vi "rszvl_core_global.vi"() -> ()   [LabVIEW 2014] (continued)
 Callback"="", "Supported Models"="", "Instrument Options"="", "Repeated Capabilities"="", "Restricted Repeated Capabilities"="", "Help"="This attribute switches measurements with a power sensor on or off.\n\nAvailable Repeated Capabilities:\nNone\n\nRemote-control command(s):\n[SENSe<1|2>:]PMETer[:STATe] ON | OFF", "Flags"={"OPC Wait"=FALSE, "Dont check status"=FALSE, "*WAI"=FALSE}, "Check Status Callback"=""}, {"Level"=3, "Descriptive Name"="PWM Averaging State", "Class Only"=FALSE, "Data Type"=3, "Access"=2, "Identifier"="RSZVL_ATTR_PMET_AVERAGE_AUTO", "Range Table"="", "Command"="SENS:PMET:MTIM:AVER:STAT", "Read Callback"="", "Write Callback"="", "Range Callback"="", "Check Callback"="", "Rngtable Callback"="", "Coerce Callback"="", "User Callback"="", "Supported Models"="", "Instrument Options"="", "Repeated Capabilities"="", "Restricted Repeated Capabilities"="", "Help"="This attribute activates or deactivates manual averaging. The average count is set with the [SENSe<1|2>:]PMETer:MTIMe:AVERage:COUNt command (RSZVL_ATTR_PMET_AVERAGE_COUNT attribute).\n\nAvailable Repeated Capabilities:\nNone\n\nRemote-control command(s):\n[SENSe<1|2>:]PMETer:MTIMe:AVERage[:STATe] ON | OFF", "Flags"={"OPC Wait"=FALSE, "Dont check status"=FALSE, "*WAI"=FALSE}, "Check Status Callback"=""}, {"Level"=3, "Descriptive Name"="PWM Averaging Count", "Class Only"=FALSE, "Data Type"=0, "Access"=2, "Identifier"="RSZVL_ATTR_PMET_AVERAGE_COUNT", "Range Table"="rszvl_rngPmetAverCount", "Command"="SENS:PMET:MTIM:AVER:COUN", "Read Callback"="", "Write Callback"="", "Range Callback"="", "Check Callback"="", "Rngtable Callback"="", "Coerce Callback"="", "User Callback"="", "Supported Models"="", "Instrument Options"="", "Repeated Capabilities"="", "Restricted Repeated Capabilities"="", "Help"="This attribute defines the number of readings (averagings) to be performed after a single sweep has been started. This attribute is only available if the [SENSe<1|2>:]PMETer:MTIMe:AVERage[:STATe] command (RSZVL_ATTR_PMET_AVERAGE_AUTO attribute) is set to ON. Results become more stable with extended average, particularly if signals with low power are measured. This setting can be used to minimize the influence of noise in the power meter measurement.\n\nAvailable Repeated Capabilities:\nNone\n\nRemote-control command(s):\n[SENSe<1|2>:]PMETer:MTIMe:AVERage:COUNt", "Flags"={"OPC Wait"=FALSE, "Dont check status"=FALSE, "*WAI"=FALSE}, "Check Status Callback"=""}, {"Level"=3, "Descriptive Name"="PWM Reference Level Offset State", "Class Only"=FALSE, "Data Type"=3, "Access"=2, "Identifier"="RSZVL_ATTR_PMET_REF_LEVEL_OFFSET_STATE", "Range Table"="", "Command"="SENS:PMET:ROFF:STAT", "Read Callback"="", "Write Callback"="", "Range Callback"="", "Check Callback"="", "Rngtable Callback"="", "Coerce Callback"="", "User Callback"="", "Supported Models"="", "Instrument Options"="", "Repeated Capabilities"="", "Restricted Repeated Capabilities"="", "Help"="This attribute defines whether the reference level offset set for the analyzer is taken into account for the measured power or not.\n\nAvailable Repeated Capabilities:\nNone\n\nRemote-control command(s):\n[SENSe<1|2>:]PMETer:ROFFset[:STATe] ON | OFF", "Flags"={"OPC Wait"=FALSE, "Dont check status"=FALSE, "*WAI"=FALSE}, "Check Status Callback"=""}, {"Level"=2, "Descriptive Name"="Display", "Class Only"=TRUE, "Data Type"=0, "Access"=0, "Identifier"="", "Range Table"="", "Command"="", "Read Callback"="", "Write Callback"="", "Range Callback"="", "Check Callback"="", "Rngtable Callback"="", "Coerce Callback"="", "User Callback"="", "Supported Models"="", "Instrument Options"="", "Repeated Capabilities"="", "Restricted Repeated Capabilities"="", "Help"="(1) PWM Result Display:\nThis attribute switches bargraph display on or off for measurements with a power sensor. If bargraph display is switched off, the measurement value appears in the Marker Info field.\n\n(2) PWM Rel/Abs Display:\nThis attribute switches between relative and absolute display of the result.", "Flags"={"OPC Wait"=FALSE, "Dont check status"=FALSE, "*WAI"=FALSE}, "Check Status Callback"=""}, {"Level"=3, "Descriptive Name"="PWM Rel/Abs Display", "Class Only"=FALSE, "Data Type"=3, "Access"=2, "Identifier"="RSZVL_ATTR_PMET_RELATIVE", "Range Table"="", "Command"="CALC:PMET:REL:STAT", "Read Callback"="", "Write Callback"="", "Range Callback"="", "Check Callback"="", "Rngtable Callback"="", "Coerce Callback"="", "User Callback"="", "Supported Models"="", "Instrument Options"="", "Repeated Capabilities"="", "Restricted Repeated Capabilities"="", "Help"="This attribute switches between relative and absolute display of the result.\n\nAvailable Repeated Capabilities:\nNone\n\nRemote-control command(s):\nCALCulate<1|2>:PMETer:RELative:STATe ON | OFF", "Flags"={"OPC Wait"=FALSE, "Dont check status"=FALSE, "*WAI"=FALSE}, "Check Status Callback"=""}, {"Level"=2, "Descriptive Name"="Results", "Class Only"=TRUE, "Data Type"=0, "Access"=0, "Identifier"="", "Range Table"="", "Command"="", "Read Callback"="", "Write Callback"="", "Range Callback"="", "Check Callback"="", "Rngtable Callback"="", "Coerce Callback"="", "User Callback"="", "Supported Models"="", "Instrument Options"="", "Repeated Capabilities"="", "Restricted Repeated Capabilities"="", "Help"="(1) PWM Read Result:\nThis attribute triggers a measurement with the power sensor and then outputs the result.\n\n(2) PWM Fetch Result:\nThis attribute outputs the result of the power sensor.", "Flags"={"OPC Wait"=FALSE, "Dont check status"=FALSE, "*WAI"=FALSE}, "Check Status Callback"=""}, {"Level"=3, "Descriptive Name"="PWM Read Result", "Class Only"=FALSE, "Data Type"=1, "Access"=0, "Identifier"="RSZVL_ATTR_PMET_READ", "Range Table"="", "Command"="READ:PMET?", "Read Callback"="", "Write Callback"="", "Range Callback"="", "Check Callback"="", "Rngtable Callback"="", "Coerce Callback"="", "User Callback"="", "Supported Models"="", "Instrument Options"="", "Repeated Capabilities"="", "Restricted Repeated Capabilities"="", "Help"="This attribute triggers a measurement with the power sensor and then outputs the result.\n\nAvailable Repeated Capabilities:\nNone\n\nRemote-control command(s):\nREAD<1|2>:PMETer?", "Flags"={"OPC Wait"=TRUE, "Dont check status"=FALSE, "*WAI"=FALSE}, "Check Status Callback"=""}, {"Level"=3, "Descriptive Name"="PWM Fetch Result", "Class Only"=FALSE, "Data Type"=1, "Access"=0, "Identifier"="RSZVL_ATTR_PMET_FETCH", "Range Table"="", "Command"="FETC:PMET?", "Read Callback"="", "Write Callback"="", "Range Callback"="", "Check Callback"="", "Rngtable Callback"="", "Coerce Callback"="", "User Callback"="", "Supported Models"="", "Instrument Options"="", "Repeated Capabilities"="", "Restricted Repeated Capabilities"="", "Help"="This attribute outputs the result of the power sensor.\n\nAvailable Repeated Capabilities:\nNone\n\nRemote-control command(s):\nFETCh<1|2>:PMETer?", "Flags"={"OPC Wait"=FALSE, "Dont check status"=FALSE, "*WAI"=FALSE}, "Check Status Callback"=""}, {"Level"=1, "Descriptive Name"="K14 - Spectrogram Measurement", "Class Only"=TRUE, "Data Type"=0, "Access"=0, "Identifier"="", "Range Table"="", "Command"="", "Read Callback"="", "Write Callback"="", "Range Callback"="", "Check Callback"="", "Rngtable Callback"="", "Coerce Callback"="", "User Callback"="", "Supported Models"="", "Instrument Options"="", "Repeated Capabilities"="", "Restricted Repeated Capabilities"="", "Help"="This class contains attributes for the Spectrogram Measurement option (K14).\n\n(1) Settings (Class):\nAttributes that configure Spectrogram.\n\n(2) Marker Settings (Class):\nAttributes that configure markers for Spectrogram.", "Flags"={"OPC Wait"=FALSE, "Dont check status"=FALSE, "*WAI"=FALSE}, "Check Status Callback"=""}, {"Level"=2, "Descriptive Name"="Settings", "Class Only"=TRUE, "Data Type"=0, "Access"=0, "Identifier"="", "Range Table"="", "Command"="", "Read Callback"="", "Write Callback"="", "Range Callback"="", "Check Callback"="", "Rngtable Callback"="", "Coerce Callback"="", "User Callback"="", "Supported Models"="", "Instrument Options"="", "Repeated Capabilities"="", "Restricted Repeated Capabilities"="", "Help"="Attributes that configure Spectrogram.\n\n(1) Spectrogram State:\nThis attribute activates or deactivates the Spectrogram Measurement option.\n\n(2) Spectrogram Color:\nThis attribute defines the frame color setting.\n\n(3) Spectrogram Display Size:\nThis attribute changes the screen layout.\n\n(4) Spectrogram History Buffer:\nThis attribute sets the number of frames to be stored in the history buffer.\n\n(5) Spectrogram Time Stamp:\nThis attribute activates or deactivates the time stamp.\n\n(6) Spectrogram Frame Count:\nThis attribute sets the number of frames recorded in a single sweep measurement.\n\n(7) Spectrogram Frame Select:\nThis attribute selects the frame if no measurement is running. During a measurement, the value is fixed to 0 and this command is not available.\n\n(8) Spectrogram Continue Frame:\nThis attribute determines whether the results of the last measurement are deleted before starting a new measurement in single sweep mode.\n\n(9) Spectrogram Clear:\nThis attribute deletes the spectrogram result display and the history buffer.\n\n(10) Spectrogram File Items to Save Recall Spectrogram:\nThis attribute adds the spectrogram data to the list of data subsets of a save/recall device setting.", "Flags"={"OPC Wait"=FALSE, "Dont check status"=FALSE, "*WAI"=FALSE}, "Check Status Callback"=""}, {"Level"=3, "Descriptive Name"="Spectrogram State", "Class Only"=FALSE, "Data Type"=3, "Access"=2, "Identifier"="RSZVL_ATTR_SPEM_STATE", "Range Table"="", "Command"="CALC:SPEC", "Read Callback"="", "Write Callback"="", "Range Callback"="", "Check Callback"="", "Rngtable Callback"="", "Coerce Callback"="", "User Callback"="", "Supported Models"="", "Instrument Options"="", "Repeated Capabilities"="", "Restricted Repeated Capabilities"="", "Help"="This attribute activates or deactivates the Spectrogram Measurement option.\n\nAvailable Repeated Capabilities:\nNone\n\nRemote-control command(s):\nCALCulate<1|2>:SPECtrogram[:STATe] OFF | ON", "Flags"={"OPC Wait"=FALSE, "Dont check status"=FALSE, "*WAI"=FALSE}, "Check Status Callback"=""}, {"Level"=3, "Descriptive Name"="Spectrogram Color", "Class Only"=FALSE, "Data Type"=0, "Access"=2, "Identifier"="RSZVL_ATTR_SPEM_COLOR", "Range Table"="rszvl_rngSpemColor", "Command"="CALC:SPEC:COL", "Read Callback"="", "Write Callback"="", "Range Callback"="", "Check Callback"="", "Rngtable Callback"="", "Coerce Callback"="", "User Callback"="", "Supported Models"="", "Instrument Options"="", "Repeated Capabilities"="", "Restricted Repeated Capabilities"="", "Help"="This attribute defines the frame color setting.\n\nAvailable Repeated Capabilities:\nNone\n\nRemote-control command(s):\nCALCulate<1|2>:SPECtrogram:COLor", "Flags"={"OPC Wait"=FALSE, "Dont check status"=FALSE, "*WAI"=FALSE}, "Check Status Callback"=""}, {"Level"=3, "Descriptive Name"="Spectrogram Display Size", "Class Only"=FALSE, "Data Type"=0, "Access"=2, "Identifier"="RSZVL_ATTR_SPEM_SIZE", "Range Table"="rszvl_rngDISPSizeWindow", "Command"="CALC:SPEC:SIZE", "Read Callback"="", "Write Callback"="", "Range Callback"="", "Check Callback"="", "Rngtable Callback"="", "Coerce Callback"="", "User Callback"="", "Supported Models"="", "Instrument Options"="", "Repeated Capabilities"="", "Restricted Repeated Capabilities"="", "Help"="This attribute changes the screen layout.\n\nAvailable Repeated Capabilities:\nNone\n\nRemote-control command(s):\nCALCulate<1|2>:SPECtrogram:SIZE", "Flags"={"OPC Wait"=FALSE, "Dont check status"=FALSE, "*WAI"=FALSE}, "Check Status Callback"=""}, {"Level"=3, "Descriptive Name"="Spectrogram History Buffer", "Class Only"=FALSE, "Data Type"=0, "Access"=2, "Identifier"="RSZVL_ATTR_SPEM_HDEP", "Range Table"="rszvl_rngSpemHistoryBuffDepth", "Command"="CALC:SPEC:HDEP", "Read Callback"="", "Write Callback"="", "Range Callback"="", "Check Callback"="", "Rngtable Callback"="", "Coerce Callback"="", "User Callback"="", "Supported Models"="", "Instrument Options"="", "Repeated Capabilities"="", "Restricted Repeated Capabilities"="", "Help"="This attribute sets the number of frames to be stored in the history buffer.\n\nAvailable Repeated Capabilities:\nNone\n\nRemote-control command(s):\nCALCulate<1|2>:SPECtrogram:HDEPth", "Flags"={"OPC Wait"=FALSE, "Dont check status"=FALSE, "*WAI"=FALSE}, "Check Status Callback"=""}, {"Level"=3, "Descriptive Name"="Spectrogram Time Stamp", "Class Only"=FALSE, "Data Type"=3, "Access"=2, "Identifier"="RSZVL_ATTR_SPEM_TIME_STAMP_STATE", "Range Table"="", "Command"="CALC:SPEC:TST", "Read Callback"="", "Write Callback"="", "Range Callback"="", "Check Callback"="", "Rngtable Callback"="", "Coerce Callback"="", "User Callback"="", "Supported Models"="", "Instrument Options"="", "Repeated Capabilities"="", "Restricted Repeated Capabilities"="", "Help"="This attribute activates or deactivates the time stamp.\n\nAvailable Repeated Capabilities:\nNone\n\nRemote-control command(s):\nCALCulate<1|2>:SPECtrogram:TSTamp[:STATe]", "Flags"={"OPC Wait"=FALSE, "Dont check status"=FALSE, "*WAI"=FALSE}, "Check Status Callback"=""}, {"Level"=3, "Descriptive Name"="Spectrogram Frame Count", "Class Only"=FALSE, "Data Type"=0, "Access"=2, "Identifier"="RSZVL_ATTR_SPEM_FRAME_COUNT", "Range Table"="", "Command"="CALC:SPEC:FRAM:COUN", "Read Callback"="", "Write Callback"="", "Range Callback"="", "Check Callback"="", "Rngtable Callback"="", "Coerce Callback"="", "User Callback"="", "Supported Models"="", "Instrument Options"="", "Repeated Capabilities"="", "Restricted Repeated Capabilities"="", "Help"="This attribute sets the number of frames recorded in a single sweep measurement.\n\nAvailable Repeated Capabilities:\nNone\n\nRemote-control command(s):\nCALCulate<1|2>:SPECtrogram:FRAMe:COUNt", "Flags"={"OPC Wait"=FALSE, "Dont check status"=FALSE, "*WAI"=FALSE}, "Check Status Callback"=""}, {"Level"=3, "Descriptive Name"="Spectrogram Frame Select", "Class Only"=FALSE, "Data Type"=0, "Access"=2, "Identifier"="RSZVL_ATTR_SPEM_FRAME_SELECT", "Range Table"="", "Command"="CALC:SPEC:FRAM:SEL", "Read Callback"="", "Write Callback"="", "Range Callback"="", "Check Callback"="", "Rngtable Callback"="", "Coerce Callback"="", "User Callback"="", "Supported Models"="", "Instrument Options"="", "Repeated Capabilities"="", "Restricted Repeated Capabilities"="", "Help"="This attribute selects the frame if no measurement is running. During a measurement, the value is fixed to 0 and this command is not available.\n\nAvailable Repeated Capabilities:\nNone\n\nRemote-control command(s):\nCALCulate<1|2>:SPECtrogram:FRAMe:SELect", "Flags"={"OPC Wait"=FALSE, "Dont check status"=FALSE, "*WAI"=FALSE}, "Check Status Callback"=""}, {"Level"=3, "Descriptive Name"="Spectrogram Continue Frame", "Class Only"=FALSE, "Data Type"=3, "Access"=2, "Identifier"="RSZVL_ATTR_SPEM_CONTINUOUS", "Range Table"="", "Command"="CALC:SPEC:CONT", "Read Callback"="", "Write Callback"="", "Range Callback"="", "Check Callback"="", "Rngtable Callback"="", "Coerce Callback"="", "User Callback"="", "Supported Models"="", "Instrument Options"="", "Repeated Capabilities"="", "Restricted Repeated Capabilities"="", "Help"="This attribute determines whether the results of the last measurement are deleted before starting a new measurement in single sweep mode.\n\nAvailable Repeated Capabilities:\nNone\n\nRemote-control command(s):\nCALCulate<1|2>:SPECtrogram:CONTinuous ON | OFF", "Flags"={"OPC Wait"=FALSE, "Dont check status"=FALSE, "*WAI"=FALSE}, "Check Status Callback"=""}, {"Level"=3, "Descriptive Name"="Spectrogram Clear", "Class Only"=FALSE, "Data Type"=4, "Access"=1, "Identifier"="RSZVL_ATTR_SPEM_CLEAR", "Range Table"="", "Command"="CALC:SPEC:CLE", "Read Callback"="", "Write Callback"="", "Range Callback"="", "Check Callback"="", "Rngtable Callback"="", "Coerce Callback"="", "User Callback"="", "Supported Models"="", "Instrument Options"="", "Repeated Capabilities"="", "Restricted Repeated Capabilities"="", "Help"="This attribute deletes the spectrogram result display and the history buffer.\n\nAvailable Repeated Capabilities:\nNone\n\nRemote-control command(s):\nCALCulate<1|2>:SPECtrogram:CLEar[:IMMediate]", "Flags"={"OPC Wait"=FALSE, "Dont check status"=FALSE, "*WAI"=FALSE}, "Check Status Callback"=""}, {"Level"=3, "Descriptive Name"="Spectrogram File Items to Save Recall Spectrogram", "Class Only"=FALSE, "Data Type"=3, "Access"=2, "Identifier"="RSZVL_ATTR_FILE_ITEMS_SAVE_RECAL_SPEM", "Range Table"="", "Command"="MMEM:SEL:SPEC", "Read Callback"="", "Write Callback"="", "Range Callback"="", "Check Callback"="", "Rngtable Callback"="", "Coerce Callback"="", "User Callback"="", "Supported Models"="", "Instrument Options"="", "Repeated Capabilities"="", "Restricted Repeated Capabilities"="", "Help"="This attribute adds the spectrogram data to the list of data subsets of a save/recall device setting.\n\nAvailable Repeated Capabilities:\nNone\n\nRemote-control command(s):\nMMEMory:SELect[:ITEM]:SPECtrogram ON | OFF", "Flags"={"OPC Wait"=FALSE, "Dont check status"=FALSE, "*WAI"=FALSE}, "Check Status Callback"=""}, {"Level"=2, "Descriptive Name"="Marker Settings", "Class Only"=TRUE, "Data Type"=0, "Access"=0, "Identifier"="", "Range Table"="", "Command"="", "Read Callback"="", "Write Callback"="", "Range Callback"="", "Check Callback"="", "Rngtable Callback"="", "Coerce Callback"="", "User Callback"="", "Supported Models"="", "Instrument Options"="", "Repeated Capabilities"="", "Restricted Repeated Capabilities"="", "Help"="Attributes that configure markers for Spectrogram.\n\n\n(1) Spectrogram Marker Frame Number:\nThis attribute defines the frame number of the specified marker.\n\n(2) Spectrogram Marker Search Area:\nThis attribute defines the search area of the specified marker.\n\n(3) Spectrogram Marker Search XY:\nThis attribute positions the specified marker on the current minimum or maximum of the search area.\n\n(4) Spectrogram Marker Search Y:\nThis attribute positions the specified marker on the current maximum/minimum, next maximu/minimum above or belove in y–axis direction (constant x–axis value).\n\n(5) Spectrogram Delta Marker Frame Number:\nThis attribute defines the frame number of the specified delta marker.\n\n(6) Spectrogram Delta Marker Search Area:\nThis attribute defines the search area of the specified delta marker.\n\n(7) Spectrogram Delta Marker Search XY:\nThis attribute positions the specified delta marker on the current maximum of the search area.\n\n(8) Spectrogram Delta Marker Search Y:\nThis attribute positions the specified delta marker on the current maximum/minimum, next maximu/minimum above or belove in y–axis direction (constant x–axis value).", "Flags"={"OPC Wait"=FALSE, "Dont check status"=FALSE, "*WAI"=FALSE}, "Check Status Callback"=""}, {"Level"=3, "Descriptive Name"="Spectrogram Marker Frame Number", "Class Only"=FALSE, "Data Type"=0, "Access"=2, "Identifier"="RSZVL_ATTR_SPEM_MARK_FRAME_NUMBER", "Range Table"="", "Command"="CALC:MARK{Marker}:SPEC:FRAM", "Read Callback"="", "Write Callback"="", "Range Callback"="", "Check Callback"="", "Rngtable Callback"="", "Coerce Callback"="", "User Callback"="", "Supported Models"="", "Instrument Options"="", "Repeated Capabilities"="", "Restricted Repeated Capabilities"="", "Help"="This attribute defines the frame number of the specified marker.\n\nAvailable Repeated Capabilities:\nMarker: M1,M2,M3,M4\r\n\nRemote-control command(s):\nCALCulate<1|2>:MARKer<1...4>:SPECtrogram:FRAMe", "Flags"={"OPC Wait"=FALSE, "Dont check status"=FALSE, "*WAI"=FALSE}, "Check Status Callback"=""}, {"Level"=3, "Descriptive Name"="Spectrogram Marker Search Area", "Class Only"=FALSE, "Data Type"=0, "Access"=2, "Identifier"="RSZVL_ATTR_SPEM_MARKER_SEARCH_AREA", "Range Table"="rszvl_rngSpemSearchArea", "Command"="CALC:MARK{Marker}:SPEC:SAR", "Read Callback"="", "Write Callback"="", "Range Callback"="", "Check Callback"="", "Rngtable Callback"="", "Coerce Callback"="", "User Callback"="", "Supported Models"="", "Instrument Options"="", "Repeated Capabilities"="", "Restricted Repeated Capabilities"="", "Help"="This attribute defines the search area of the specified marker.\n\nAvailable Repeated Capabilities:\nMarker: M1,M2,M3,M4\r\n\nRemote-control command(s):\nCALCulate<1|2>:MARKer<1...4>:SPECtrogram:SARea", "Flags"={"OPC Wait"=FALSE, "Dont check status"=FALSE, "*WAI"=FALSE}, "Check Status Callback"=""}, {"Level"=3, "Descriptive Name"="Spectrogram Marker Search XY", "Class Only"=FALSE, "Data Type"=4, "Access"=1, "Identifier"="RSZVL_ATTR_SPEM_MARKER_SEARCH_XY", "Range Table"="", "Command"="CALC:MARK{Marker}:SPEC:XY:{ModifMinMaxAver}", "Read Callback"="", "Write Callback"="", "Range Callback"="", "Check Callback"="", "Rngtable Callback"="", "Coerce Callback"="", "User Callback"="", "Supported Models"="", "Instrument Options"="", "Repeated Capabilities"="", "Restricted Repeated Capabilities"="", "Help"="This attribute positions the specified marker on the current minimum or maximum of the search area.\n\nAvailable Repeated Capabilities:\nMarker: M1,M2,M3,M4\r\nModifMinMaxAver: Min,Max,Aver\r\n\nRemote-control command(s):\nCALCulate<1|2>:MARKer<1...4>:SPECtrogram:XY:<MAXimum[:PEAK] | MINimum[:PEAK]>", "Flags"={"OPC Wait"=FALSE, "Dont check status"=FALSE, "*WAI"=FALSE}, "Check Status Callback"=""}, {"Level"=3, "Descriptive Name"="Spectrogram Marker Search Y", "Class Only"=FALSE, "Data Type"=4, "Access"=1, "Identifier"="RSZVL_ATTR_SPEM_MARKER_SEARCH_Y", "Range Table"="", "Command"="CALC:MARK{Marker}:SPEC:Y:{ModifMinMaxAver}:{ModifAboveBelow}", "Read Callback"="", "Write Callback"="", "Range Callback"="", "Check Callback"="", "Rngtable Callback"="", "Coerce Callback"="", "User Callback"="", "Supported Models"="", "Instrument Options"="", "Repeated Capabilities"="", "Restricted Repeated Capabilities"="", "Help"="This attribute positions the specified marker on the current maximum/minimum, next maximu/minimum above or belove in y–axis direction (constant x–axis value).\n\nAvailable Repeated Capabilities:\nMarker: M1,M2,M3,M4\r\nModifMinMaxAver: Min,Max,Aver\r\nModifAboveBelow: Peak,Above,Below,Next\r\n\nRemote-control command(s):\nCALCulate<1|2>:MARKer<1...4>:SPECtrogram:Y:<MAXimum | MINimum>:<[PEAK] | ABOVe | BELow | NEXT>", "Flags"={"OPC Wait"=FALSE, "Dont check status"=FALSE, "*WAI"=FALSE}, "Check Status Callback"=""}, {"Level"=3, "Descriptive Name"="Spectrogram Delta Marker Frame Number", "Class Only"=FALSE, "Data Type"=0, "Access"=2, "Identifier"="RSZVL_ATTR_SPEM_DELT_FRAME_NUMBER", "Range Table"="", "Command"="CALC:DELT{DeltaMarker}:SPEC:FRAM", "Read Callback"="", "Write Callback"="", "Range Callback"="", "Check Callback"="", "Rngtable Callback"="", "Coerce Callback"="", "User Callback"="", "Supported Models"="", "Instrument Options"="", "Repeated Capabilities"="", "Restricted Repeated Capabilities"="", "Help"="This attribute defines the frame number of the specified delta marker.\n\nAvailable Repeated Capabilities:\nDeltaMarker: DM1,DM2,DM3,DM4\r\n\nRemote-control command(s):\nCALCulate<1|2>:DELTamarkerer<1...4>:SPECtrogram:FRAMe", "Flags"={"OPC Wait"=FALSE, "Dont check status"=FALSE, "*WAI"=FALSE}, "Check Status Callback"=""}, {"Level"=3, "Descriptive Name"="Spectrogram Delta Marker Search Area", "Class Only"=FALSE, "Data Type"=0, "Access"=2, "Identifier"="RSZVL_ATTR_SPEM_DELT_SEARCH_AREA", "Range Table"="rszvl_rngSpemSearchArea", "Command"="CALC:DELT{DeltaMarker}:SPEC:SAR", "Read Callback"="", "Write Callback"="", "Range Callback"="", "Check Callback"="", "Rngtable Callback"="", "Coerce Callback"="", "User Callback"="", "Supported Models"="", "Instrument Options"="", "Repeated Capabilities"="", "Restricted Repeated Capabilities"="", "Help"="This attribute defines the search area of the specified delta marker.\n\nAvailable Repeated Capabilities:\nDeltaMarker: DM1,DM2,DM3,DM4\r\n\nRemote-control command(s):\nCALCulate<1|2>:DELTamarker<1...4>:SPECtrogram:SARea", "Flags"={"OPC Wait"=FALSE, "Dont check status"=FALSE, "*WAI"=FALSE}, "Check Status Callback"=""}, {"Level"=3, "Descriptive Name"="Spectrogram Delta Marker Search XY", "Class Only"=FALSE, "Data Type"=4, "Access"=1, "Identifier"="RSZVL_ATTR_SPEM_DELT_SEARCH_XY", "Range Table"="", "Command"="CALC:DELT{DeltaMarker}:SPEC:XY:{ModifMinMaxAver}", "Read Callback"="", "Write Callback"="", "Range Callback"="", "Check Callback"="", "Rngtable Callback"="", "Coerce Callback"="", "User Callback"="", "Supported Models"="", "Instrument Options"="", "Repeated Capabilities"="", "Restricted Repeated Capabilities"="", "Help"="This attribute positions the specified delta marker on the current maximum of the search area.\n\nAvailable Repeated Capabilities:\nDeltaMarker: DM1,DM2,DM3,DM4\r\nModifMinMaxAver: Min,Max,Aver\r\n\nRemote-control command(s):\nCALCulate<1|2>:DELTamarker<1...4>:SPECtrogram:XY:<MAXimum | MINimum>[:PEAK]", "Flags"={"OPC Wait"=FALSE, "Dont check status"=FALSE, "*WAI"=FALSE}, "Check Status Callback"=""}, {"Level"=3, "Descriptive Name"="Spectrogram Delta Marker Search Y", "Class Only"=FALSE, "Data Type"=4, "Access"=1, "Identifier"="RSZVL_ATTR_SPEM_DELT_SEARCH_Y", "Range Table"="", "Command"="CALC:DELT{DeltaMarker}:SPEC:Y:{ModifMinMaxAver}:{ModifAboveBelow}", "Read Callback"="", "Write Callback"="", "Range Callback"="", "Check Callback"="", "Rngtable Callback"="", "Coerce Callback"="", "User Callback"="", "Supported Models"="", "Instrument Options"="", "Repeated Capabilities"="", "Restricted Repeated Capabilities"="", "Help"="This attribute positions the specified delta marker on the current maximum/minimum, next maximu/minimum above or belove in y–axis direction (constant x–axis value).\n\nAvailable Repeated Capabilities:\nDeltaMarker: DM1,DM2,DM3,DM4\r\nModifMinMaxAver: Min,Max,Aver\r\nModifAboveBelow: Peak,Above,Below,Next\r\n\nRemote-control command(s):\nCALCulate<1|2>:DELTamarkerer<1...4>:SPECtrogram:Y:<MAXimum | MINimum>:<[PEAK] | ABOVe | BELow | NEXT>", "Flags"={"OPC Wait"=FALSE, "Dont check status"=FALSE, "*WAI"=FALSE}, "Check Status Callback"=""}, {"Level"=1, "Descriptive Name"="K20 - Cable TV Measurements", "Class Only"=TRUE, "Data Type"=0, "Access"=0, "Identifier"="", "Range Table"="", "Command"="", "Read Callback"="", "Write Callback"="", "Range Callback"="", "Check Callback"="", "Rngtable Callback"="", "Coerce Callback"="", "User Callback"="", "Supported Models"="", "Instrument Options"="", "Repeated Capabilities"="", "Restricted Repeated Capabilities"="", "Help"="This class contain attributes for the Cable TV Measurement option (K20).\n\n(1) Settings (Class):\nAttributes that configure common settings of Cable TV measurement.\n\n(2) ATV Settings (Class):\nAttributes that configure ATV Settings.\n\n(3) ATV Limit Settings (Class):\nAttributes that configure ATV Limit Settings.\n\n(4) ATV Limit Results (Class):\nAttributes that return ATV limit results.\n\n\n(5) ATV Results (Class):\nAttributes that return ATV measurement results.\n\n(6) DTV Settings (Class):\nAttributes that configure DTV Settings.\n\n(7) DTV Limit Settings (Class):\nAttributes that configure DTV Limit Settings.\n\n(8) DTV Limit Results (Class):\nAttributes that return DTV limit results.\n\n(9) DTV Results (Class):\nAttributes that return DTV measurement results.\n\n(10) TV Analyzer Settings (Class):\nAttributes that configure TV Analyzer Settings.", "Flags"={"OPC Wait"=FALSE, "Dont check status"=FALSE, "*WAI"=FALSE}, "Check Status Callback"=""}, {"Level"=2, "Descriptive Name"="Settings", "Class Only"=TRUE, "Data Type"=0, "Access"=0, "Identifier"="", "Range Table"="", "Command"="", "Read Callback"="", "Write Callback"="", "Range Callback"="", "Check Callback"="", "Rngtable Callback"="", "Coerce Callback"="", "User Callback"="", "Supported Models"="", "Instrument Options"="", "Repeated Capabilities"="", "Restricted Repeated Capabilities"="", "Help"="Attributes that configure common settings of Cable TV measurement.\n\n(1) CATV Mode:\nThis attribute sets the Cable TV Measurements operating mode.\n\n(2) CATV Y Axis Auto Scaling:\nThis attribute activates the automatic scaling for the Hum and Tilt measurement. If activated, the scaling is automatically optimized to the best display of data. This rescaling may affect the values of any of the parameters under the SCALe node.\n\n(3) CATV Echo Pattern Zoom State:\nThis attribute activates or deactivates the zoom on around 0 Us for the Echo Pattern measurement.\n\n(4) CATV Echo Pattern Zoom Factor:\nThis attribute sets the zoom factor for the Echo Pattern measurement.\n\n(5) CATV Modulation Error Zoom:\nThis attribute sets the zoom for the Modulation Errors measurement.\n\n(6) CATV Overview Zoom:\nThis attribute sets the zoom for the Overview measurement.\n\n(7) CATV Constellation Diagram Zoom:\nThis attribute sets the zoom for the constellation diagram.\n\n(8) CATV Constellation Diagram Display Mode :\nThis attribute sets the display mode of the constallation diagram.\n\n(9) CATV Measurement Channel:\nThis attribute defines the active measurement channel.\n\n(10) CATV RF Frequency:\nThis attribute defines the RF frequency. The interpretation of the RF frequency depends on the signal type. For details refer to chapter \"Instrument Functions\", section \"Cable TV Measurement Option (K20)\", RF softkey.\n\n(11) CATV RF Frequency Step Size:\nThis attribute configures TV channel frequency step size.\n\n(12) CATV Frequency Axis Labeling:\nThis attribute defines the labeling of the frequency axis.\n\n(13) CATV Side Band:\nThis attribute defines the sideband position.\n\n(14) CATV Modulation Standard:\nThis attribute defines the name for a modulation standard.\n\n(15) CATV Modulation Standard Group Delay:\nThis attribute defines the group delay for a modulation standard.\n\n(16) CATV Modulation Standard Signal Type:\nThis attribute defines the signal type of a modulation standard.", "Flags"={"OPC Wait"=FALSE, "Dont check status"=FALSE, "*WAI"=FALSE}, "Check Status Callback"=""}, {"Level"=3, "Descriptive Name"="CATV Mode", "Class Only"=FALSE, "Data Type"=4, "Access"=1, "Identifier"="RSZVL_ATTR_CATV_MODE", "Range Table"="", "Command"="INST:SEL CATV", "Read Callback"="", "Write Callback"="", "Range Callback"="", "Check Callback"="", "Rngtable Callback"="", "Coerce Callback"="", "User Callback"="", "Supported Models"="", "Instrument Options"="", "Repeated Capabilities"="", "Restricted Repeated Capabilities"="", "Help"="This attribute sets the Cable TV Measurements operating mode.\n\nAvailable Repeated Capabilities:\nNone\n\nRemote-control command(s):\nINSTrument:SELect CATV", "Flags"={"OPC Wait"=FALSE, "Dont check status"=FALSE, "*WAI"=FALSE}, "Check Status Callback"=""}, {"Level"=3, "Descriptive Name"="CATV Y Axis Auto Scaling", "Class Only"=FALSE, "Data Type"=4, "Access"=1, "Identifier"="RSZVL_ATTR_CATV_Y_SCALE_AUTO", "Range Table"="", "Command"="DISP:TRAC:Y:AUTO", "Read Callback"="", "Write Callback"="", "Range Callback"="", "Check Callback"="", "Rngtable Callback"="", "Coerce Callback"="", "User Callback"="", "Supported Models"="", "Instrument Options"="", "Repeated Capabilities"="", "Restricted Repeated Capabilities"="", "Help"="This attribute activates the automatic scaling for the Hum and Tilt measurement. If activated, the scaling is automatically optimized to the best display of data. This rescaling may affect the values of any of the parameters under the SCALe node.\n\nAvailable Repeated Capabilities:\nNone\n\nRemote-control command(s):\nDISPlay[:WINDow<1|2>]:TRACe<1...4>:Y[:SCALe]:AUTO", "Flags"={"OPC Wait"=FALSE, "Dont check status"=FALSE, "*WAI"=FALSE}, "Check Status Callback"=""}, {"Level"=3, "Descriptive Name"="CATV Echo Pattern Zoom State", "Class Only"=FALSE, "Data Type"=3, "Access"=2, "Identifier"="RSZVL_ATTR_CATV_EPAT_ZOOM_STATE", "Range Table"="", "Command"="DISP:ZOOM:EPAT:STAT", "Read Callback"="", "Write Callback"="", "Range Callback"="", "Check Callback"="", "Rngtable Callback"="", "Coerce Callback"="", "User Callback"="", "Supported Models"="", "Instrument Options"="", "Repeated Capabilities"="", "Restricted Repeated Capabilities"="", "Help"="This attribute activates or deactivates the zoom on around 0 Us for the Echo Pattern measurement.\n\nAvailable Repeated Capabilities:\nNone\n\nRemote-control command(s):\nDISPlay[:WINDow<1|2>]:ZOOM:STATe ON | OFF", "Flags"={"OPC Wait"=FALSE, "Dont check status"=FALSE, "*WAI"=FALSE}, "Check Status Callback"=""}, {"Level"=3, "Descriptive Name"="CATV Echo Pattern Zoom Factor", "Class Only"=FALSE, "Data Type"=0, "Access"=2, "Identifier"="RSZVL_ATTR_CATV_EPAT_ZOOM_FACTOR", "Range Table"="rszvl_rngCatvEpattZoom", "Command"="DISP:ZOOM:EPAT", "Read Callback"="", "Write Callback"="", "Range Callback"="", "Check Callback"="", "Rngtable Callback"="", "Coerce Callback"="", "User Callback"="", "Supported Models"="", "Instrument Options"="", "Repeated Capabilities"="", "Restricted Repeated Capabilities"="", "Help"="This attribute sets the zoom factor for the Echo Pattern measurement.\n\nAvailable Repeated Capabilities:\nNone\n\nRemote-control command(s):\nDISPlay[:WINDow<1|2>]:ZOOM:EPATtern", "Flags"={"OPC Wait"=FALSE, "Dont check status"=FALSE, "*WAI"=FALSE}, "Check Status Callback"=""}, {"Level"=3, "Descriptive Name"="CATV Modulation Error Zoom", "Class Only"=FALSE, "Data Type"=0, "Access"=2, "Identifier"="RSZVL_ATTR_CATV_MERR_ZOOM", "Range Table"="rszvl_rngCatvMerrZoom", "Command"="DISP:ZOOM:MERR", "Read Callback"="", "Write Callback"="", "Range Callback"="", "Check Callback"="", "Rngtable Callback"="", "Coerce Callback"="", "User Callback"="", "Supported Models"="", "Instrument Options"="", "Repeated Capabilities"="", "Restricted Repeated Capabilities"="", "Help"="This attribute sets the zoom for the Modulation Errors measurement.\n\nAvailable Repeated Capabilities:\nNone\n\nRemote-control command(s):\nDISPlay[:WINDow<1|2>]:ZOOM:MERRors NONE | IMBalance | QERRor | SUPpression | PJITter | MERRms | MERPeak | EVMRms | EVMPeak", "Flags"={"OPC Wait"=FALSE, "Dont check status"=FALSE, "*WAI"=FALSE}, "Check Status Callback"=""}, {"Level"=3, "Descriptive Name"="CATV Overview Zoom", "Class Only"=FALSE, "Data Type"=0, "Access"=2, "Identifier"="RSZVL_ATTR_CATV_OVER_ZOOM", "Range Table"="rszvl_rngCatvOverZoom", "Command"="DISP:ZOOM:OVER", "Read Callback"="", "Write Callback"="", "Range Callback"="", "Check Callback"="", "Rngtable Callback"="", "Coerce Callback"="", "User Callback"="", "Supported Models"="", "Instrument Options"="", "Repeated Capabilities"="", "Restricted Repeated Capabilities"="", "Help"="This attribute sets the zoom for the Overview measurement.\n\nAvailable Repeated Capabilities:\nNone\n\nRemote-control command(s):\nDISPlay[:WINDow<1|2>]:ZOOM:OVERview NONE | MERRms | MERPeak | EVMRms | EVMPeak | CFOFfset | SROFfset", "Flags"={"OPC Wait"=FALSE, "Dont check status"=FALSE, "*WAI"=FALSE}, "Check Status Callback"=""}, {"Level"=3, "Descriptive Name"="CATV Constellation Diagram Zoom", "Class Only"=FALSE, "Data Type"=0, "Access"=2, "Identifier"="RSZVL_ATTR_CATV_QUAD_ZOOM", "Range Table"="rszvl_rngCatvConstDiagZoom", "Command"="DISP:ZOOM:QUAD", "Read Callback"="", "Write Callback"="", "Range Callback"="", "Check Callback"="", "Rngtable Callback"="", "Coerce Callback"="", "User Callback"="", "Supported Models"="", "Instrument Options"="", "Repeated Capabilities"="", "Restricted Repeated Capabilities"="", "Help"="This attribute sets the zoom for the constellation diagram.\n\nAvailable Repeated Capabilities:\nNone\n\nRemote-control command(s):\nDISPlay[:WINDow<1|2>]:ZOOM:QUADrant NONE | 1 | 2 | 3 | 4", "Flags"={"OPC Wait"=FALSE, "Dont check status"=FALSE, "*WAI"=FALSE}, "Check Status Callback"=""}, {"Level"=3, "Descriptive Name"="CATV Constellation Diagram Display Mode", "Class Only"=FALSE, "Data Type"=3, "Access"=2, "Identifier"="RSZVL_ATTR_CATV_TRACE_MODE_FREEZE", "Range Table"="", "Command"="DISP:TRAC{Trace}:MODE:FRE", "Read Callback"="", "Write Callback"="", "Range Callback"="", "Check Callback"="", "Rngtable Callback"="", "Coerce Callback"="", "User Callback"="", "Supported Models"="", "Instrument Options"="", "Repeated Capabilities"="", "Restricted Repeated Capabilities"="", "Help"="This attribute sets the display mode of the constallation diagram.\n\nAvailable Repeated Capabilities:\nTrace: TR1,TR2,TR3,TR4,TR5,TR6,TR7,TR8,TR9,TR10,TR11,TR12,TR13,TR14,TR15,TR16,TR17,TR18,TR19,TR20\r\n\nRemote-control command(s):\nDISPlay[:WINDow<1|2>]:TRACe<1...4>:MODE:FREeze[:STATe]", "Flags"={"OPC Wait"=FALSE, "Dont check status"=FALSE, "*WAI"=FALSE}, "Check Status Callback"=""}, {"Level"=3, "Descriptive Name"="CATV Measurement Channel", "Class Only"=FALSE, "Data Type"=0, "Access"=2, "Identifier"="RSZVL_ATTR_CATV_CHANNEL", "Range Table"="", "Command"="FREQ:CHAN", "Read Callback"="", "Write Callback"="", "Range Callback"="", "Check Callback"="", "Rngtable Callback"="", "Coerce Callback"="", "User Callback"="", "Supported Models"="", "Instrument Options"="", "Repeated Capabilities"="", "Restricted Repeated Capabilities"="", "Help"="This attribute defines the active measurement channel.\n\nAvailable Repeated Capabilities:\nNone\n\nRemote-control command(s):\n[SENSe<1|2>:]FREQuency:CHANnel", "Flags"={"OPC Wait"=FALSE, "Dont check status"=FALSE, "*WAI"=FALSE}, "Check Status Callback"=""}, {"Level"=3, "Descriptive Name"="CATV RF Frequency", "Class Only"=FALSE, "Data Type"=1, "Access"=2, "Identifier"="RSZVL_ATTR_CATV_RF_FREQUENCY", "Range Table"="rszvl_rngCatvRFFreq", "Command"="FREQ:RF", "Read Callback"="", "Write Callback"="", "Range Callback"="", "Check Callback"="", "Rngtable Callback"="", "Coerce Callback"="", "User Callback"="", "Supported Models"="", "Instrument Options"="", "Repeated Capabilities"="", "Restricted Repeated Capabilities"="", "Help"="This attribute defines the RF frequency. The interpretation of the RF frequency depends on the signal type. For details refer to chapter \"Instrument Functions\", section \"Cable TV Measurement Option (K20)\", RF softkey.\n\nAvailable Repeated Capabilities:\nNone\n\nRemote-control command(s):\n[SENSe<1|2>:]FREQuency:RF", "Flags"={"OPC Wait"=FALSE, "Dont check status"=FALSE, "*WAI"=FALSE}, "Check Status Callback"=""}, {"Level"=3, "Descriptive Name"="CATV RF Frequency Step Size", "Class Only"=FALSE, "Data Type"=1, "Access"=2, "Identifier"="RSZVL_ATTR_CATV_RF_FREQUENCY_STEP_SIZE", "Range Table"="", "Command"="FREQ:STEP", "Read Callback"="", "Write Callback"="", "Range Callback"="", "Check Callback"="", "Rngtable Callback"="", "Coerce Callback"="", "User Callback"="", "Supported Models"="", "Instrument Options"="", "Repeated Capabilities"="", "Restricted Repeated Capabilities"="", "Help"="This attribute configures TV channel frequency step size.\n\nAvailable Repeated Capabilities:\nNone\n\nRemote-control command(s):\n[SENSe<1|2>:]FREQuency:STEP", "Flags"={"OPC Wait"=FALSE, "Dont check status"=FALSE, "*WAI"=FALSE}, "Check Status Callback"=""}, {"Level"=3, "Descriptive Name"="CATV Frequency Axis Labeling", "Class Only"=FALSE, "Data Type"=0, "Access"=2, "Identifier"="RSZVL_ATTR_CATV_SWEEP_SPACING", "Range Table"="rszvl_rngAbsRel", "Command"="SWE:SPAC", "Read Callback"="", "Write Callback"="", "Range Callback"="", "Check Callback"="", "Rngtable Callback"="", "Coerce Callback"="", "User Callback"="", "Supported Models"="", "Instrument Options"="", "Repeated Capabilities"="", "Restricted Repeated Capabilities"="", "Help"="This attribute defines the labeling of the frequency axis.\n\nAvailable Repeated Capabilities:\nNone\n\nRemote-control command(s):\n[SENSe<1|2>:]SWEep:SPACing", "Flags"={"OPC Wait"=FALSE, "Dont check status"=FALSE, "*WAI"=FALSE}, "Check Status Callback"=""}, {"Level"=3, "Descriptive Name"="CATV Side Band", "Class Only"=FALSE, "Data Type"=0, "Access"=2, "Identifier"="RSZVL_ATTR_CATV_SIDE_BAND", "Range Table"="rszvl_rngCatvSBand", "Command"=":DDEM:SBAN", "Read Callback"="", "Write Callback"="", "Range Callback"="", "Check Callback"="", "Rngtable Callback"="", 
